vi "Event Text For Check Registration.vi"(10 "hotel to check":string, 11 "guests":set{string}(c389)) -> (3 "message":string)   [LabVIEW 2023]
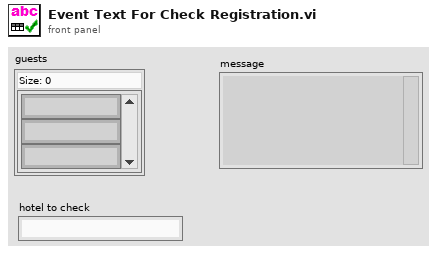
[diagram p1: front panel]
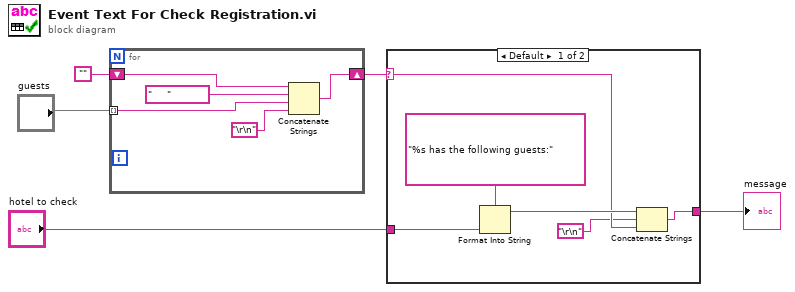
[diagram p0: block diagram]
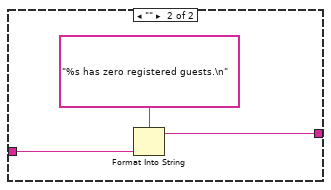
[diagram p2: hidden frame]
diagram:
  n1 = for {
    tunnel: "guests" -> [w9] mode=indexing
    shift-right: [w10] -> w3
    shift-left: "" -> [w8]
    n2 = Concatenate Strings(w8, "     ", w9, "\r\n") -> (w10:string)
  }
  n3 = case shown="Default" w3 {
    selector: w3 -> [w13 _]
    tunnel: "hotel to check" -> [w15 w18]
    tunnel: [w11 w17] -> w5
    frame Default {
      n4 = Format Into String(format string="%s has the following guests:" ("L10n_message 2"), w15) -> (resulting string=w14:string)  [unwired: 2 in, 1 out]
      n5 = Concatenate Strings(w14, "\r\n", w13) -> (w11:string)
    }
    frame "" {
      n6 = Format Into String(format string="%s has zero registered guests.\n" ("L10n_message 1"), w18) -> (resulting string=w17:string)  [unwired: 2 in, 1 out]
    }
  }
  "message" <- w5
